vi "terminate.vi"(8 "error in (no error)":errorcluster, 11 "DAQ_DL091205Readers in":refnum<class "DAQ_DL091205Readers.lvclass">) -> (0 "error out":errorcluster, 3 "DAQ_DL091205Readers out":refnum<class "DAQ_DL091205Readers.lvclass">)   [LabVIEW 2010, in "DAQ_DL091205Readers.lvclass"]
doc: "The dynamic dispatch version of this VI terminates the plug-in object by releasing all of its resources."
uses:
  DAQ_DL091205Readers.lvclass
  DAQ_DL091205Readers.lvclass/DAQ_DL091205Readers.ctl
  SignalReader/GenericSignalReader/GenericSignalReader/GenericSignalReader.lvclass
  DAQ_DL090211Scaffold/DAQ_DL090211Scaffold/DAQ_DL090211Scaffold.lvclass
  common/classes/ErrorController/ErrorController/class_data.vi
  common/classes/ErrorController/ErrorController/ErrorController.lvclass
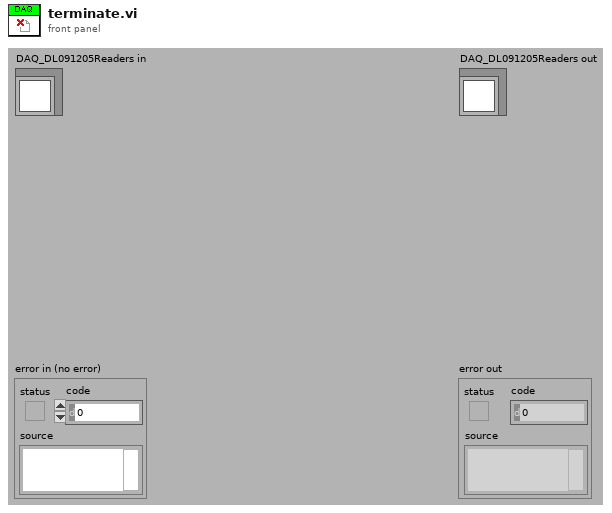
[diagram p1: front panel]
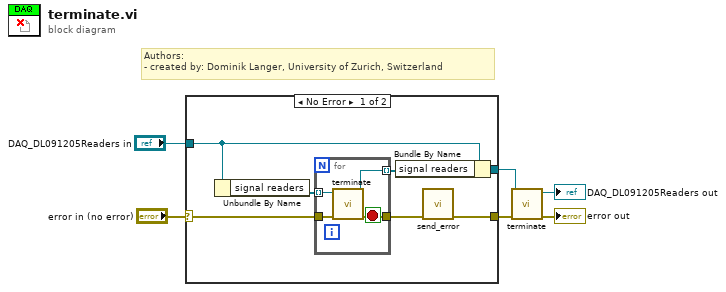
[diagram p0: block diagram]
diagram:
  # "Authors: \n- created by: Dominik Langer, University of Zurich, Switzerland"
  n1 = case shown="No Error" "error in (no error)" {
    selector: "error in (no error)" -> [w9 w18]
    tunnel: [w8 w18] -> w4
    tunnel: "DAQ_DL091205Readers in" -> [w13 w19]
    tunnel: [w12 w19] -> w2
    frame No Error {
      n2 = Unbundle By Name(w13) -> ("signal readers"=w11:refnum<class "GenericSignalReader.lvclass">[])
      n3 = for {
        tunnel: w11 -> [w17] mode=indexing
        tunnel: [w15] -> w10 mode=indexing
        tunnel: w9 -> [w16]
        tunnel: [w14] -> w7
        stop <- w14 stop-if-true
        n4 = call-dynamic "terminate.vi"("error in (no error)"=w16, "GenericPlugin in"=w17) -> ("error out"=w14:errorcluster, "GenericPlugin out"=w15:refnum<class "GenericSignalReader.lvclass">)  [unwired: 8 in]
      }
      n5 = Bundle By Name(cluster=w13, "signal readers"=w10) -> (w12:refnum<class "DAQ_DL091205Readers.lvclass">)
      n6 = call "send_error.vi"("error in (no error)"=w7) -> ("error out"=w8:errorcluster)  [unwired: 10 in]
    }
    frame Error {
    }
  }
  n7 = call-parent "terminate.vi"("error in (no error)"=w4, "GenericPlugin in"=w2) -> ("error out"=→"error out":errorcluster, "GenericPlugin out"=→"DAQ_DL091205Readers out":refnum<class "DAQ_DL091205Readers.lvclass">)  [unwired: 8 in]
